vi "test.vi"   [LabVIEW 2016]
uses:
  Instrument_Setup.vi
types:
  T1 = cluster{"GPIB address":i16, "GPIB bus":i16, "connection ID":refnum<k5>, "IP":string, "Active Comm Interface":u16, "Serial Port":refnum<visa-resource-name>, "Programmer Type":u16, "TCP Port y":dbl}
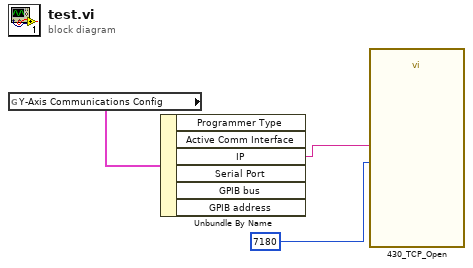
[diagram p0: block diagram]
diagram:
  n1 = global read "Instrument_Setup.vi" "Y-Axis Communications Config"() -> (w3:T1)
  n2 = Unbundle By Name(w3) -> ("IP"=w2:string)  [unwired: 5 out]
  n3 = call "430_TCP_Open.vi"("IP Address"=w2, "TCP Port"=7180) -> ()  [unwired: 4 in, 3 out]
